vi "Create Status.vi"(8 "error in (no error)":errorcluster, 11 "Historian Logger in":refnum<class "Historian Logger.lvclass">) -> (0 "error out":errorcluster, 2 "Logger Status":T1, 3 "Historian Logger out":refnum<class "Historian Logger.lvclass">)   [LabVIEW 2020, in "VolatusHistorian.lvlib" / "Historian Logger.lvclass"]
uses:
  Historian Logger.lvclass
  Historian Logger.lvclass/Historian Logger.ctl
  Logger Status.ctl
  VolatusHistorian.lvlib
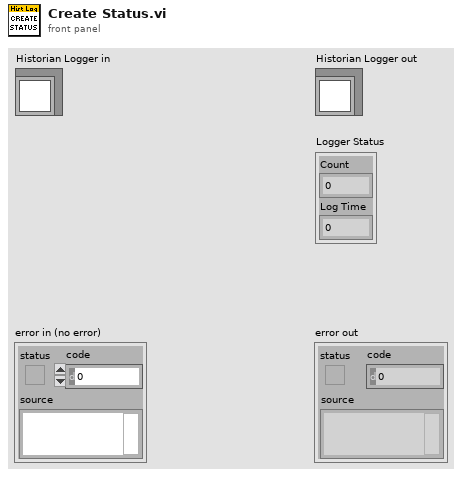
[diagram p1: front panel]
types:
  T1 = typedef "VolatusHistorian.lvlib/Logger Status.ctl" = cluster{"Count":i32, "Log Time":dbl}
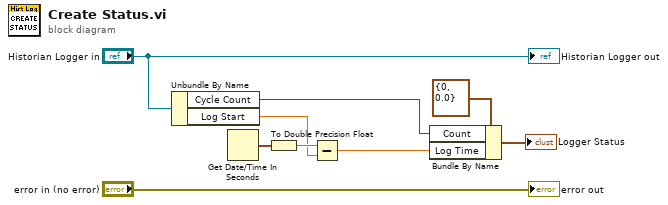
[diagram p0: block diagram]
diagram:
  n1 = Unbundle By Name("Historian Logger in") -> ("Cycle Count"=w5:i32, "Log Start"=w2:dbl)
  n2 = Get Date/Time In Seconds() -> (seconds since 1Jan1904=w4:timestamp)
  n3 = To Double Precision Float(number=w4) -> (double precision float=w3:dbl)
  n4 = Subtract(x=w3, y=w2) -> (x-y=w1:dbl)
  n5 = Bundle By Name(cluster=T1 {"Count"=0, "Log Time"=0.0} ("Logger Status"), "Count"=w5, "Log Time"=w1) -> (→"Logger Status":T1)
  "error out" <- "error in (no error)"
  "Historian Logger out" <- "Historian Logger in"
